vi "Prueba_acelerometro.vi"() -> ()   [LabVIEW 2025]
panel:
  in  "Calibrar":bool
  out "3D Picture":refnum<vi>(3d-picture)
  out "Z":u16
  out "Y":u16
  out "X":u16
  in  "VISA resource name":refnum<visa-resource-name>
  out "error out":errorcluster
  in  "stop":bool
  in  "Color":u32(colorbox)
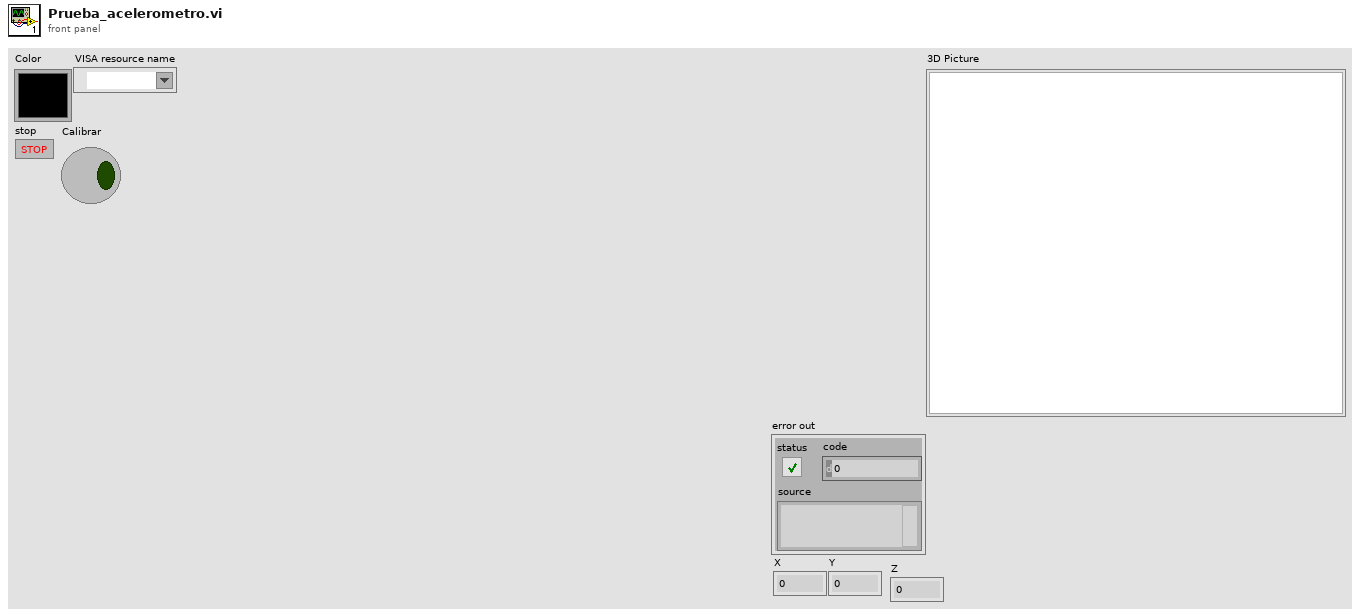
[diagram p1: front panel]
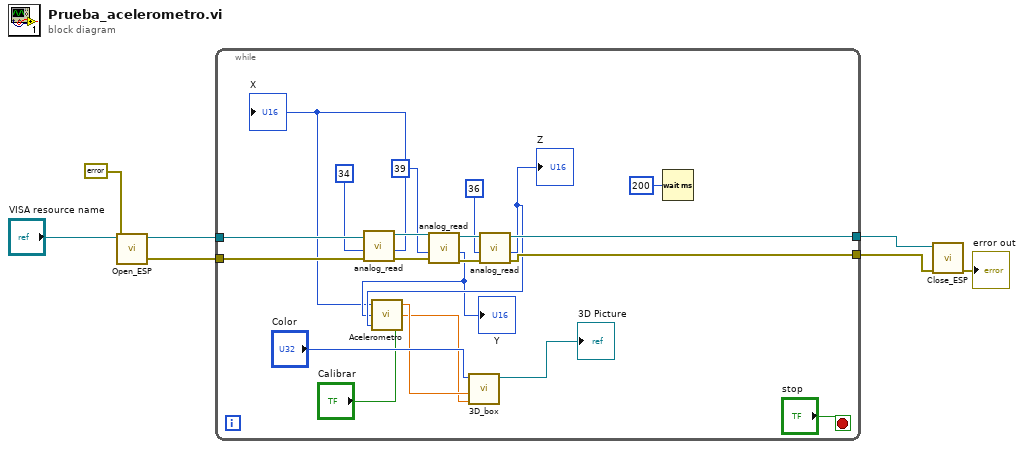
[diagram p0: block diagram]
diagram:
  n1 = call "Open_ESP.vi"("error in (no error)"=errorcluster {"status"=FALSE, "code"=0, "source"=""}, "VISA resource name"="VISA resource name") -> ("error out"=w6:errorcluster, "VISA resource name out"=w5:refnum<visa-resource-name>)  [unwired: 8 in]
  n2 = while {
    tunnel: [w24] -> w7
    tunnel: w6 -> [w22]
    tunnel: w5 -> [w21]
    tunnel: [w16] -> w4
    stop <- "stop" stop-if-true
    n3 = call "analog_read.vi"("error in (no error)"=w22, "Pin"=u8 34, "VISA resource name"=w21) -> ("error out"=w23:errorcluster, "Analog read"=w8:u16, "VISA resource name out"=w20:refnum<visa-resource-name>)  [unwired: 6 in]
    "X" <- w8
    n4 = call "analog_read.vi"("error in (no error)"=w23, "Pin"=u8 39, "VISA resource name"=w20) -> ("error out"=w26:errorcluster, "Analog read"=w9:u16, "VISA resource name out"=w25:refnum<visa-resource-name>)  [unwired: 6 in]
    "Y" <- w9
    n5 = call "analog_read.vi"("error in (no error)"=w26, "Pin"=u8 36, "VISA resource name"=w25) -> ("error out"=w24:errorcluster, "Analog read"=w10:u16, "VISA resource name out"=w16:refnum<visa-resource-name>)  [unwired: 6 in]
    "Z" <- w10
    n6 = call "Acelerometro.vi"("Calibrar"="Calibrar", "Analog read Z"=w10, "Analog read Y"=w9, "Analog read X"=w8) -> ("PITCH"=w12:dbl, "ROLL"=w13:dbl)
    n7 = call "3D_box.vi"("PITCH"=w12, "ROLL"=w13, "Color"="Color") -> ("3D Picture"=→"3D Picture":refnum<vi>)  [unwired: 8 in]
    n8 = Wait (ms)(milliseconds to wait=u32 200) -> ()  [unwired: 1 out]
  }
  n9 = call "Close_ESP.vi"("error in (no error)"=w7, "VISA resource name"=w4) -> ("error out"=→"error out":errorcluster)  [unwired: 9 in]
